vi "Read Log VI.vi"(8 "error in (no error)":errorcluster, 11 "System Log in":refnum<class "System Log.lvclass">) -> (0 "error out":errorcluster, 2 "Log VI":refnum<vi>, 3 "System Log out":refnum<class "System Log.lvclass">)   [LabVIEW 2014, in "System Log.lvclass"]
uses:
  System Log.lvclass
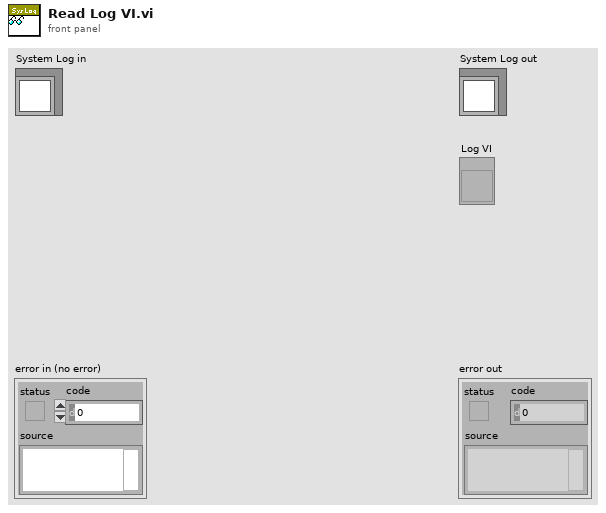
[diagram p1: front panel]
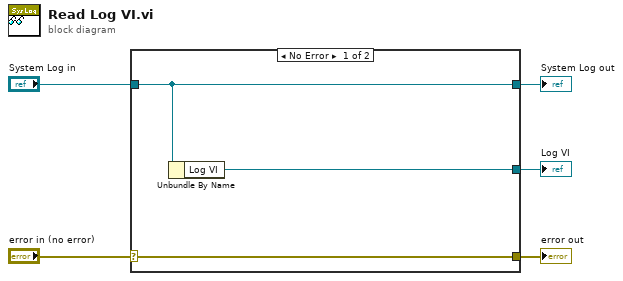
[diagram p0: block diagram]
diagram:
  n1 = case shown="No Error" "error in (no error)" {
    selector: "error in (no error)" -> [w8 w9]
    tunnel: [w8 w9] -> w4
    tunnel: [w7 w10] -> w2
    tunnel: "System Log in" -> [w7 w10]
    tunnel: [w6 _] -> w1
    frame No Error {
      n2 = Unbundle By Name(w7) -> ("Log VI"=w6:refnum<vi>)
    }
    frame Error {
    }
  }
  "error out" <- w4
  "System Log out" <- w2
  "Log VI" <- w1
